vi "Poll List.vi"(8 "error in (no error)":errorcluster, 11 "Node Ptr":T1 format="%.0x") -> (0 "error out":errorcluster)   [LabVIEW 2019, in "OPC UA Client Addon System Explorer.lvlib"]
uses:
  OPC UA Client Addon System Explorer.lvlib
  <vilib>/NI VeriStand/Custom Device API/Custom Device API.lvlib
  <vilib>/NI VeriStand/Custom Device API/Custom Device Item Ref.ctl
panel:
  out "Tags":i32(listbox)
  in  "Poll Rate (ms)":dbl
  in  "SHDocVw.IWebBrowser":refnum<k7>(container)
  in  "Header":cluster{"Section Name":string}={"Section Name"="Custom Device Item Settings"}
  in  "Description":string
  in  "Name":string
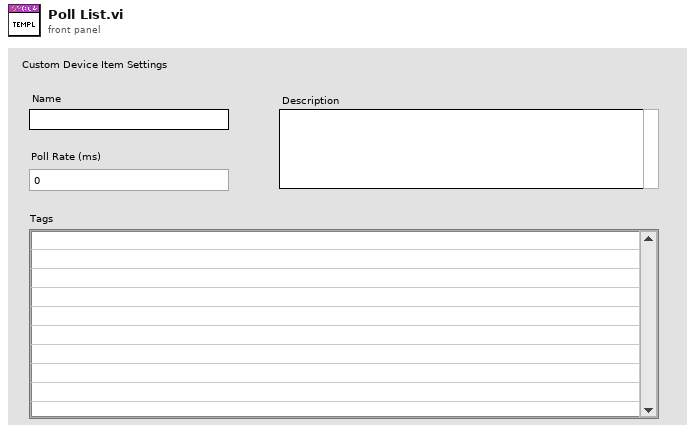
[diagram p1: front panel]
types:
  T1 = typedef "Custom Device API.lvlib/Custom Device Item Ref.ctl" = u64
  T2 = typedef "Custom Device API.lvlib/Custom Device Item Info.ctl" = cluster{"Name":string, "Is Channel":bool, "GUID":string, "Is Waveform":bool}
  T3 = typedef "Custom Device API.lvlib/Custom Device Commands.ctl" = enum16{"Default", "Item renamed", "Shutdown", "Dynamic button pressed"}
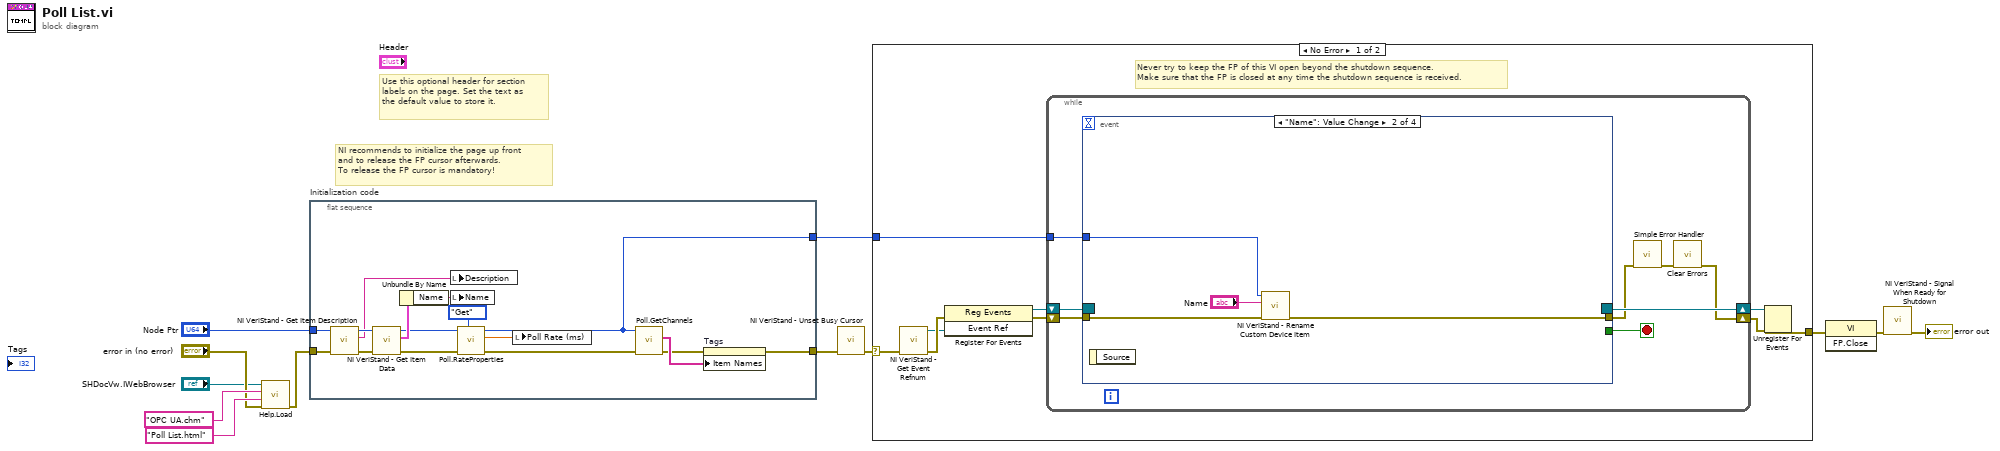
[diagram p0: block diagram]
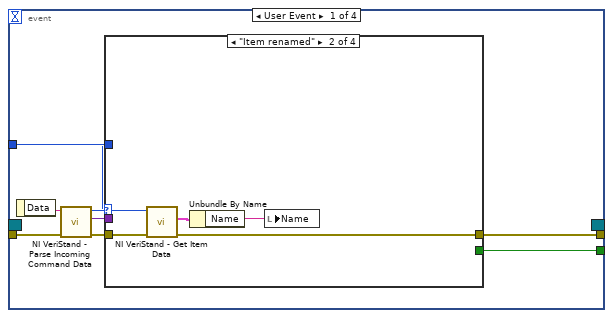
[diagram p2: hidden frame]
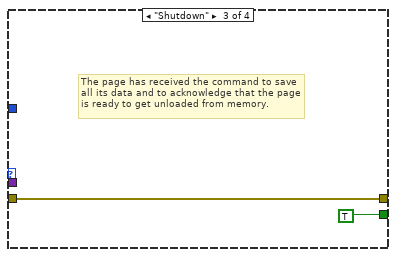
[diagram p4: hidden frame]
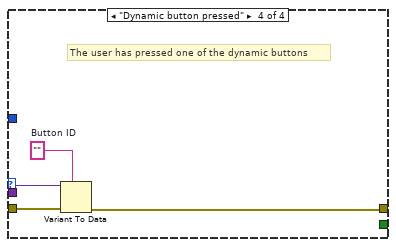
[diagram p5: hidden frame]
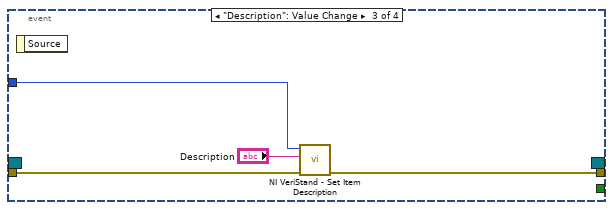
[diagram p6: hidden frame]
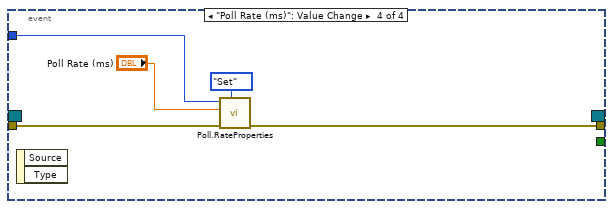
[diagram p7: hidden frame]
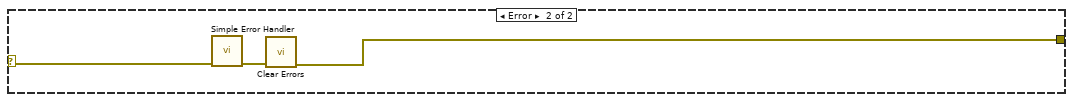
[diagram p8: hidden frame]
diagram:
  # "Use this optional header for section labels on the page. Set the text as the default value to store it."
  # "NI recommends to initialize the page up front\nand to release the FP cursor afterwards.\nTo release the FP cursor is mandatory!"
  n1 = call "Help.Load.vi"("error in (no error)"="error in (no error)", "HTML File"="Poll List.html" ("Main CHM File"), "Main CHM File"="OPC UA.chm", "SHDocVw.IWebBrowser2"="SHDocVw.IWebBrowser") -> ("error out"=w2:errorcluster)  [unwired: 7 in]
  n2 = flat-sequence "Initialization code" {
    tunnel: w2 -> [w27]
    tunnel: "Node Ptr" -> [w26]
    tunnel: [w13] -> w8
    tunnel: [w16] -> w6
    frame #0 {
      n3 = call <vilib>:"NI VeriStand - Get Item Description.vi"("error in (no error)"=w27, "Item Ref in"=w26) -> ("error out"=w24:errorcluster, "Description"=w25:string, "Item Ref out"=w28:T1)  [unwired: 7 out]
      n4 = call <vilib>:"NI VeriStand - Get Item Data.vi"("error in (no error)"=w24, "Item Ref in"=w28) -> ("error out"=w22:errorcluster, "Item Info"=w23:T2, "Item Ref out"=w21:T1)  [unwired: 7 out]
      n5 = Unbundle By Name(w23) -> ("Name"=w18:string)
      n6 = local write "Description"(w25) -> ()
      n7 = local write "Name"(w18) -> ()
      n8 = call "Poll.RateProperties.vi"("Action"=enum8{"Get", "Set"}."Get", "error in (no error)"=w22, "Item Ref in"=w21) -> ("error out"=w17:errorcluster, "Poll Rate"=w19:dbl, "Item Ref out"=w16:T1)  [unwired: 6 in]
      n9 = local write "Poll Rate (ms)"(w19) -> ()
      n10 = call "Poll.GetChannels.vi"("error in (no error)"=w17, "Node Ptr"=w16) -> ("error out"=w14:errorcluster, "Tags"=w15:string[])  [unwired: 7 in, 1 out]
      n11 = property on="Tags" class="LstBox (strict)"(error in=w14, "Item Names"=w15) -> (error out=w13:errorcluster)  [unwired: 1 in, 1 out]
    }
  }
  n12 = call <vilib>:"NI VeriStand - Unset Busy Cursor.vi"("error in (no error)"=w8) -> ("error out"=w7:errorcluster)  [unwired: 10 out]
  n13 = case shown="No Error" w7 {
    selector: w7 -> [w29 w81]
    tunnel: [w34 w79] -> w12
    tunnel: w6 -> [w30 _]
    frame No Error {
      # "Never try to keep the FP of this VI open beyond the shutdown sequence.\nMake sure that the FP is closed at any time the shutdown sequence is received."
      n14 = call <vilib>:"NI VeriStand - Get Event Refnum.vi"("error in (no error)"=w29) -> ("error out"=w37:errorcluster, "Event Ref"=w33:refnum<user-event>)  [unwired: 9 out]
      n15 = register-events(error in=w37, w33) -> (reference out=w31:refnum<event-registration>, error out=w32:errorcluster)  [unwired: 1 in]
      n16 = while {
        tunnel: w30 -> [w41]
        shift-right: [w38] -> w35
        shift-left: w32 -> [w44]
        shift-right: [w45] -> w36
        shift-left: w31 -> [w43]
        stop <- w42 stop-if-true
        n17 = event shown="[1] \"Name\": Value Change" {
          selector: w43 -> [_ _ _ _]
          dyn-events: [_ _ _ _] -> w45
          timeout: _ -> [_ _ _ _]
          tunnel: w44 -> [w53 w68 w72 w77]
          tunnel: [w49 _ _ _] -> w42
          tunnel: [w48 w67 w71 w74] -> w40
          tunnel: w41 -> [w47 w69 w73 w75]
          event User Event {
            n18 = event-data() -> ("Data"=w52:string)  [unwired: 1 out]
            n19 = call <vilib>:"NI VeriStand - Parse Incoming Command Data.vi"("error in (no error)"=w53, "Incoming data"=w52) -> ("error out"=w51:errorcluster, "Outgoing data"=w46:variant, "Action"=w50:T3)  [unwired: 7 out]
            n20 = case shown="\"Item renamed\"" w50 {
              tunnel: w51 -> [w54 w59 w60 w65]
              tunnel: [_ _ TRUE _] -> w49
              tunnel: [w54 w57 w60 w62] -> w48
              tunnel: w47 -> [_ w58 _ _]
              tunnel: w46 -> [_ _ _ w64]
              frame "Default", Default {
              }
              frame "Item renamed" {
                n21 = call <vilib>:"NI VeriStand - Get Item Data.vi"("error in (no error)"=w59, "Item Ref in"=w58) -> ("error out"=w57:errorcluster, "Item Info"=w56:T2)  [unwired: 8 out]
                n22 = Unbundle By Name(w56) -> ("Name"=w55:string)
                n23 = local write "Name"(w55) -> ()
              }
              frame "Shutdown" {
                # "The page has received the command to save all its data and to acknowledge that the page is ready to get unloaded from memory."
              }
              frame "Dynamic button pressed" {
                w63 = ""  # Button ID
                # "The user has pressed one of the dynamic buttons"
                n24 = Variant To Data(error in=w65, type=w63, Variant=w64) -> (error out=w62:errorcluster)  [unwired: 1 out]
              }
            }
          }
          event "Name": Value Change {
            n25 = event-data() -> ()  [unwired: 2 out]
            n26 = call <vilib>:"NI VeriStand - Rename Custom Device Item.vi"("error in (no error)"=w68, "New Name"="Name", "Item Ref in"=w69) -> ("error out"=w67:errorcluster)  [unwired: 6 in, 2 out]
          }
          event "Description": Value Change {
            n27 = event-data() -> ()  [unwired: 2 out]
            n28 = call <vilib>:"NI VeriStand - Set Item Description.vi"("error in (no error)"=w72, "Description"="Description", "Item Ref in"=w73) -> ("error out"=w71:errorcluster)  [unwired: 8 out]
          }
          event "Poll Rate (ms)": Value Change {
            n29 = event-data() -> ()  [unwired: 3 out]
            n30 = call "Poll.RateProperties.vi"("Action"=enum8{"Get", "Set"}."Set", "error in (no error)"=w77, "Poll Rate"="Poll Rate (ms)", "Item Ref in"=w75) -> ("error out"=w74:errorcluster)  [unwired: 5 in, 2 out]
          }
        }
        n31 = call <vilib>:"Simple Error Handler.vi"("error in (no error)"=w40) -> ("error out"=w39:errorcluster)  [unwired: 1 in, 7 out]
        n32 = call <vilib>:"Clear Errors.vi"("error in (no error)"=w39) -> ("error out"=w38:errorcluster)  [unwired: 1 in, 5 out]
      }
      n33 = Unregister For Events(event registration refnum=w36, error in=w35) -> (error out=w34:errorcluster)
    }
    frame Error {
      n34 = call <vilib>:"Simple Error Handler.vi"("error in (no error)"=w81) -> ("error out"=w80:errorcluster)  [unwired: 1 in, 7 out]
      n35 = call <vilib>:"Clear Errors.vi"("error in (no error)"=w80) -> ("error out"=w79:errorcluster)  [unwired: 1 in, 5 out]
    }
  }
  n36 = invoke class="VI" method="FP.Close"(error in=w12) -> (error out=w11:errorcluster)  [unwired: 2 in, 2 out]
  n37 = call <vilib>:"NI VeriStand - Signal When Ready for Shutdown.vi"("error in (no error)"=w11) -> ("error out"=→"error out":errorcluster)  [unwired: 10 out]
